vi "niFpga wdp fft DIF 16spc.vi"(0 "real data in":fxp<+/-,8,1>[](array[numeric])=[0.0, 0.0, 0.0, 0.0, 0.0, 0.0, 0.0, 0.0, 0.0, 0.0, 0.0, 0.0, 0.0, 0.0, 0.0, 0.0], 5 "imaginary data in":fxp<+/-,8,1>[](array[numeric])=[0.0, 0.0, 0.0, 0.0, 0.0, 0.0, 0.0, 0.0, 0.0, 0.0, 0.0, 0.0, 0.0, 0.0, 0.0, 0.0], 9 "input frame start":bool, 12 "enable":bool) -> (3 "data indices":u16[](array[numeric]), 4 "real data out":fxp<+,8,1>[](array[numeric]), 6 "imaginary data out":fxp<+,8,1>[](array[numeric]), 10 "output valid":bool, 14 "ready for frame":bool, 15 "output frame start":bool)   [LabVIEW 2017]
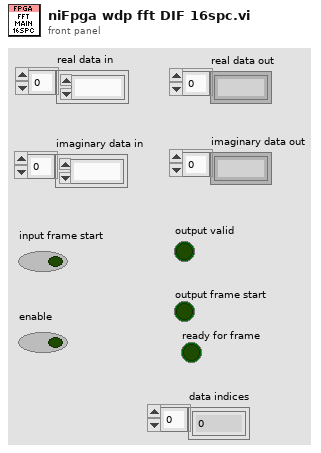
[diagram p1: front panel]
types:
  T1 = cluster{"internal input type":fxp<+/-,8,1>, "internal input type":fxp<+/-,8,1>}
  T2 = cluster{"internal input type":fxp<+/-,8,1>, "internal input type":fxp<+/-,8,1>}[]
  T3 = cluster{"x-y":fxp<+/-,20,13>, "x-y":fxp<+/-,20,13>}[]
  T4 = cluster{"data re":fxp<+/-,8,1>, "data im":fxp<+/-,8,1>}[]
  T5 = cluster{"data re":fxp<+/-,8,1>, "data im":fxp<+/-,8,1>}
  T6 = cluster{"twiddle factor type":fxp<+/-,16,2>, "twiddle factor type":fxp<+/-,16,2>}[]
  T7 = cluster{"x-y":fxp<+/-,19,12>, "x-y":fxp<+/-,19,12>}
  T8 = cluster{"x+y":fxp<+/-,19,12>, "x+y":fxp<+/-,19,12>}
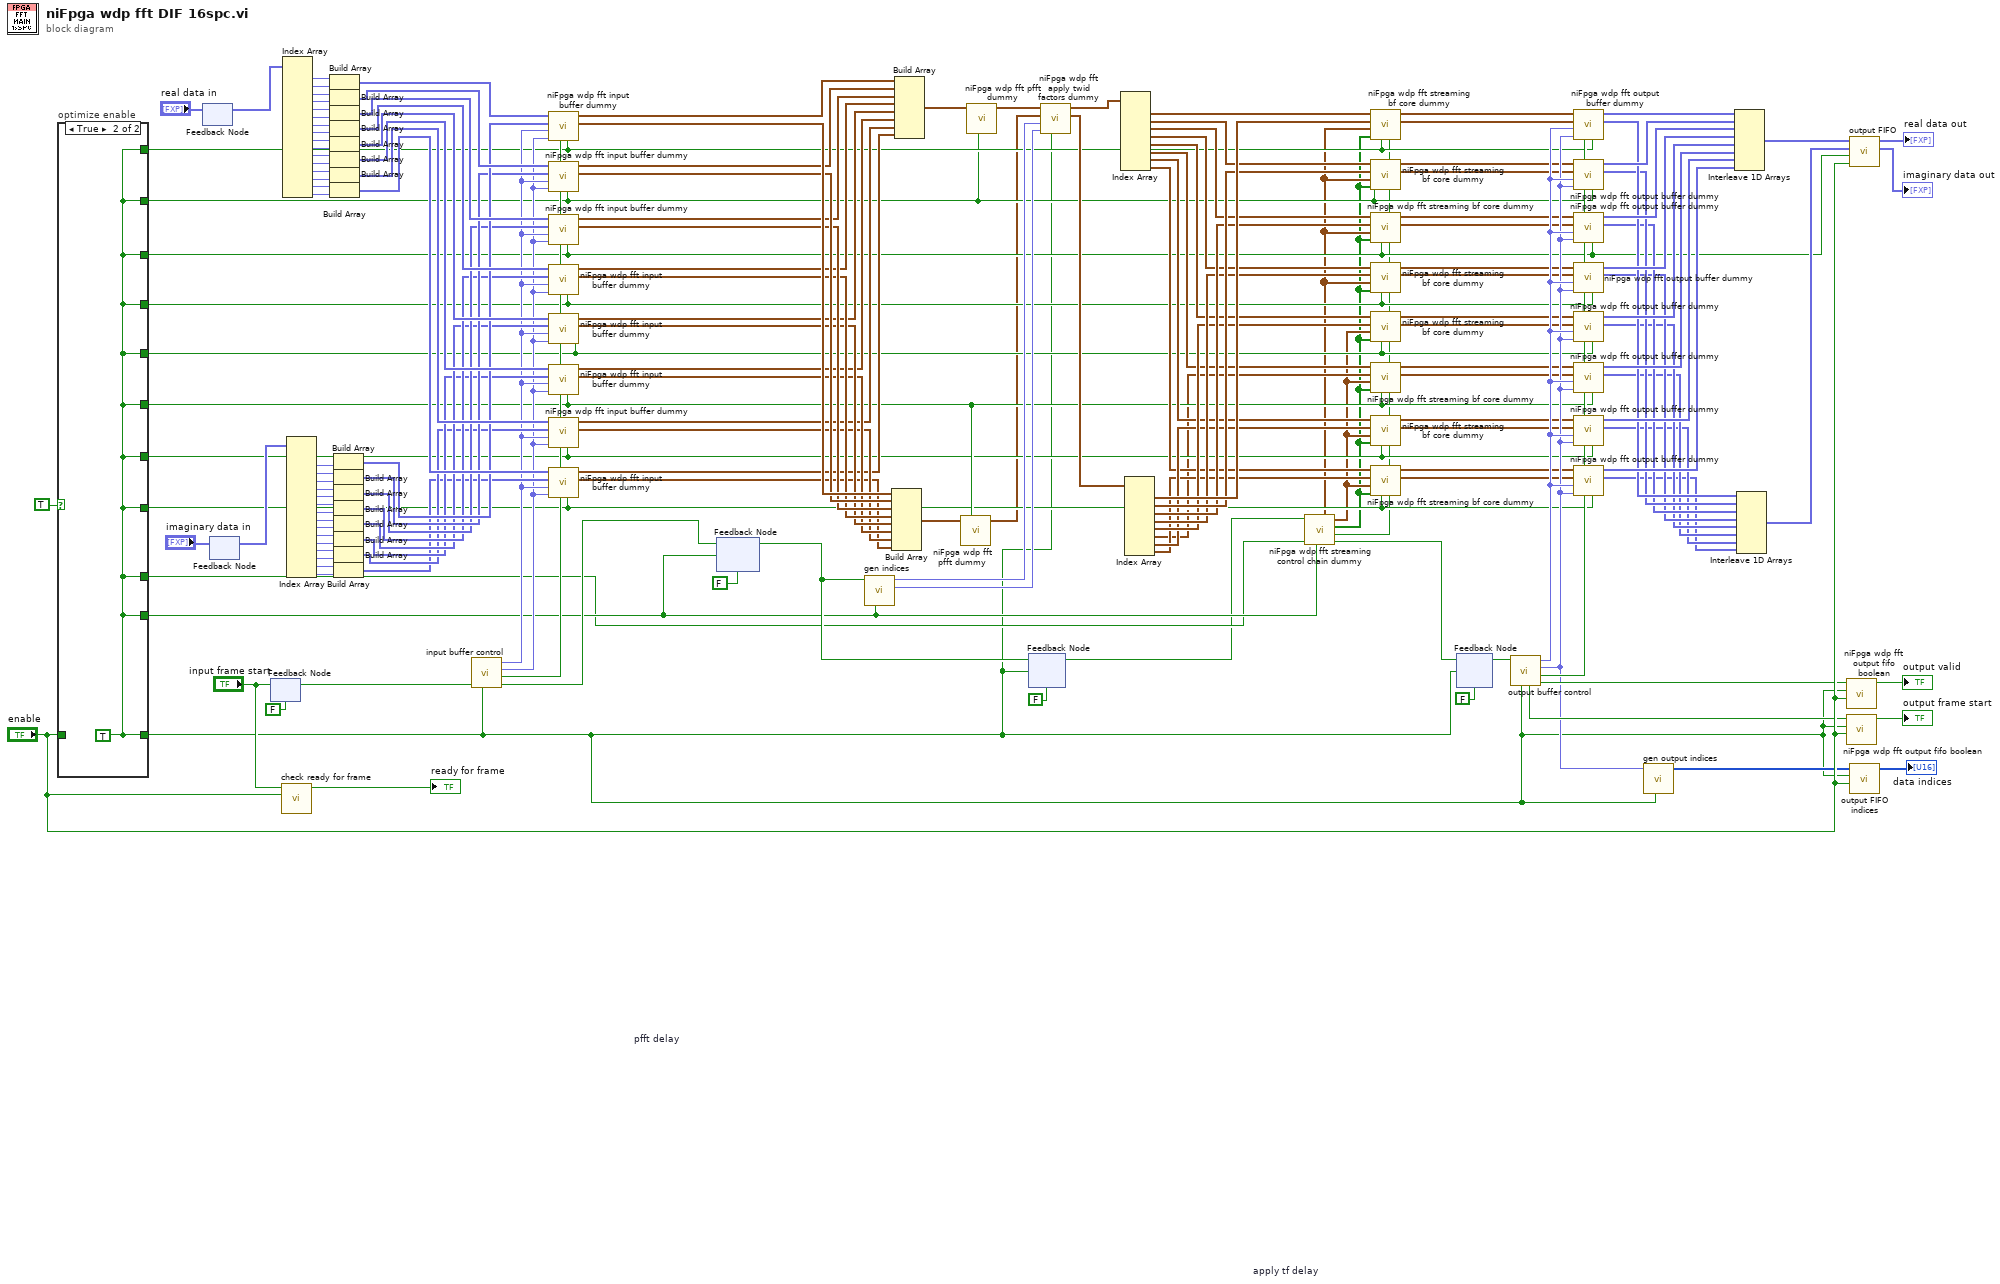
[diagram p0: block diagram]
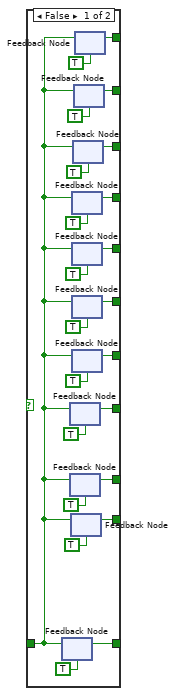
[diagram p2: hidden frame]
diagram:
  n1 = case "optimize enable" shown="True" TRUE {
    tunnel: [w191 w193] -> w41
    tunnel: [w189 w193] -> w45
    tunnel: [w180 w193] -> w57
    tunnel: [w179 w193] -> w56
    tunnel: [w178 w193] -> w55
    tunnel: [w177 w193] -> w54
    tunnel: [w176 w193] -> w53
    tunnel: [w175 w193] -> w52
    tunnel: [w174 w193] -> w51
    tunnel: [w173 w193] -> w50
    tunnel: "enable" -> [w171 _]
    tunnel: [w170 w193] -> w44
    frame False {
      n2 = feedback #1(TRUE ("enable")) -> (w191:bool)
      n3 = feedback-in #1(w171) -> ()
      n4 = feedback #2(TRUE ("enable")) -> (w173:bool)
      n5 = feedback-in #2(w171) -> ()
      n6 = feedback #3(TRUE ("enable")) -> (w170:bool)
      n7 = feedback-in #3(w171) -> ()
      n8 = feedback #4(TRUE ("enable")) -> (w189:bool)
      n9 = feedback-in #4(w171) -> ()
      n10 = feedback #5(TRUE ("enable")) -> (w177:bool)
      n11 = feedback-in #5(w171) -> ()
      n12 = feedback #6(TRUE ("enable")) -> (w176:bool)
      n13 = feedback-in #6(w171) -> ()
      n14 = feedback #7(TRUE ("enable")) -> (w175:bool)
      n15 = feedback-in #7(w171) -> ()
      n16 = feedback #8(TRUE ("enable")) -> (w174:bool)
      n17 = feedback-in #8(w171) -> ()
      n18 = feedback #9(TRUE ("enable")) -> (w178:bool)
      n19 = feedback-in #9(w171) -> ()
      n20 = feedback #10(TRUE ("enable")) -> (w179:bool)
      n21 = feedback-in #10(w171) -> ()
      n22 = feedback #11(TRUE ("enable")) -> (w180:bool)
      n23 = feedback-in #11(w171) -> ()
    }
    frame True {
      w193 = TRUE
    }
  }
  n24 = feedback #12() -> (w146:fxp<+/-,8,1>[])  [unwired: 1 in]
  n25 = feedback-in #12("real data in") -> ()
  n26 = feedback #13() -> (w137:fxp<+/-,8,1>[])  [unwired: 1 in]
  n27 = feedback-in #13("imaginary data in") -> ()
  n28 = feedback #14(FALSE ("enable")) -> (w164:bool)
  n29 = feedback-in #14("input frame start") -> ()
  n30 = call "check ready for frame"("enable"="enable", "frame start in"="input frame start") -> ("ready for frame"=→"ready for frame":bool)  [unwired: 9 in]
  n31 = Index Array(array=w146) -> (element #1=w39:fxp<+/-,8,1>, element #2=w38:fxp<+/-,8,1>, element #3=w37:fxp<+/-,8,1>, element #4=w36:fxp<+/-,8,1>, element #5=w35:fxp<+/-,8,1>, element #6=w34:fxp<+/-,8,1>, element #7=w33:fxp<+/-,8,1>, element #8=w32:fxp<+/-,8,1>, element #9=w31:fxp<+/-,8,1>, element #10=w30:fxp<+/-,8,1>, element #11=w29:fxp<+/-,8,1>, element #12=w28:fxp<+/-,8,1>, element #13=w27:fxp<+/-,8,1>, element #14=w26:fxp<+/-,8,1>, element #15=w25:fxp<+/-,8,1>, element #16=w24:fxp<+/-,8,1>)  [unwired: 16 in]
  n32 = Index Array(array=w137) -> (element #1=w8:fxp<+/-,8,1>, element #2=w9:fxp<+/-,8,1>, element #3=w10:fxp<+/-,8,1>, element #4=w11:fxp<+/-,8,1>, element #5=w12:fxp<+/-,8,1>, element #6=w13:fxp<+/-,8,1>, element #7=w14:fxp<+/-,8,1>, element #8=w15:fxp<+/-,8,1>, element #9=w16:fxp<+/-,8,1>, element #10=w17:fxp<+/-,8,1>, element #11=w18:fxp<+/-,8,1>, element #12=w19:fxp<+/-,8,1>, element #13=w20:fxp<+/-,8,1>, element #14=w21:fxp<+/-,8,1>, element #15=w22:fxp<+/-,8,1>, element #16=w23:fxp<+/-,8,1>)  [unwired: 16 in]
  n33 = Build Array(w39, w38) -> (w145:fxp<+/-,8,1>[])
  n34 = Build Array(w37, w36) -> (w144:fxp<+/-,8,1>[])
  n35 = Build Array(w35, w34) -> (w143:fxp<+/-,8,1>[])
  n36 = Build Array(w33, w32) -> (w142:fxp<+/-,8,1>[])
  n37 = Build Array(w31, w30) -> (w141:fxp<+/-,8,1>[])
  n38 = Build Array(w29, w28) -> (w140:fxp<+/-,8,1>[])
  n39 = Build Array(w27, w26) -> (w139:fxp<+/-,8,1>[])
  n40 = Build Array(w25, w24) -> (w138:fxp<+/-,8,1>[])
  n41 = Build Array(w8, w9) -> (w136:fxp<+/-,8,1>[])
  n42 = Build Array(w10, w11) -> (w135:fxp<+/-,8,1>[])
  n43 = Build Array(w12, w13) -> (w134:fxp<+/-,8,1>[])
  n44 = Build Array(w14, w15) -> (w133:fxp<+/-,8,1>[])
  n45 = Build Array(w16, w17) -> (w132:fxp<+/-,8,1>[])
  n46 = Build Array(w18, w19) -> (w131:fxp<+/-,8,1>[])
  n47 = Build Array(w20, w21) -> (w130:fxp<+/-,8,1>[])
  n48 = Build Array(w22, w23) -> (w129:fxp<+/-,8,1>[])
  n49 = call "input buffer control"("enable"=w41, "frame start in"=w164) -> ("frame start out"=w88:bool, "write memory 2?"=w121:bool, "read index"=w127:fxp<+,9,9>, "write index"=w128:fxp<+,8,8>)  [unwired: 6 in]
  n50 = call <vilib>:"niFpga wdp fft input buffer dummy.vi"("enable"=w57, "write memory 2?"=w121, "read index"=w127, "write index"=w128, "data in im"=w136, "data in re"=w145) -> ("data out 1"=w107:T1, "data out 0"=w108:T1)  [unwired: 4 in]
  n51 = call <vilib>:"niFpga wdp fft input buffer dummy.vi"("enable"=w56, "write memory 2?"=w121, "read index"=w127, "write index"=w128, "data in im"=w135, "data in re"=w144) -> ("data out 1"=w105:T1, "data out 0"=w106:T1)  [unwired: 4 in]
  n52 = call <vilib>:"niFpga wdp fft input buffer dummy.vi"("enable"=w55, "write memory 2?"=w121, "read index"=w127, "write index"=w128, "data in im"=w134, "data in re"=w143) -> ("data out 1"=w103:T1, "data out 0"=w104:T1)  [unwired: 4 in]
  n53 = call <vilib>:"niFpga wdp fft input buffer dummy.vi"("enable"=w54, "write memory 2?"=w121, "read index"=w127, "write index"=w128, "data in im"=w133, "data in re"=w142) -> ("data out 1"=w101:T1, "data out 0"=w102:T1)  [unwired: 4 in]
  n54 = call <vilib>:"niFpga wdp fft input buffer dummy.vi"("enable"=w53, "write memory 2?"=w121, "read index"=w127, "write index"=w128, "data in im"=w132, "data in re"=w141) -> ("data out 1"=w99:T1, "data out 0"=w100:T1)  [unwired: 4 in]
  n55 = call <vilib>:"niFpga wdp fft input buffer dummy.vi"("enable"=w52, "write memory 2?"=w121, "read index"=w127, "write index"=w128, "data in im"=w131, "data in re"=w140) -> ("data out 1"=w97:T1, "data out 0"=w98:T1)  [unwired: 4 in]
  n56 = call <vilib>:"niFpga wdp fft input buffer dummy.vi"("enable"=w51, "write memory 2?"=w121, "read index"=w127, "write index"=w128, "data in im"=w130, "data in re"=w139) -> ("data out 1"=w95:T1, "data out 0"=w96:T1)  [unwired: 4 in]
  n57 = call <vilib>:"niFpga wdp fft input buffer dummy.vi"("enable"=w50, "write memory 2?"=w121, "read index"=w127, "write index"=w128, "data in im"=w129, "data in re"=w138) -> ("data out 1"=w93:T1, "data out 0"=w94:T1)  [unwired: 4 in]
  n58 = feedback #15 "pfft delay"(FALSE) -> (w46:bool)
  n59 = feedback-in #15(w88, w45) -> ()
  n60 = call "gen indices"("enable"=w45, "frame start"=w46) -> ("data index 1"=w89:fxp<+,10,10>, "data index 0"=w90:fxp<+,10,10>)  [unwired: 8 in]
  n61 = Build Array(w107, w105, w103, w101, w99, w97, w95, w93) -> (w92:T2)
  n62 = Build Array(w108, w106, w104, w102, w100, w98, w96, w94) -> (w111:T2)
  n63 = call <vilib>:"niFpga wdp fft pfft dummy.vi"("enable"=w52, "data in"=w92) -> ("data out"=w5:T3)  [unwired: 9 in]
  n64 = call <vilib>:"niFpga wdp fft pfft dummy.vi"("enable"=w56, "data in"=w111) -> ("data out"=w6:T3)  [unwired: 9 in]
  n65 = feedback #16 "apply tf delay"(FALSE) -> (w40:bool)
  n66 = feedback-in #16(w46, w41) -> ()
  n67 = call <vilib>:"niFpga wdp fft apply twid factors dummy.vi"("enable"=w41, "data index 1"=w89, "data index 0"=w90, "data in 1"=w5, "data in 0"=w6) -> ("data out 1"=w109:T4, "data out 0"=w110:T4)  [unwired: 5 in]
  n68 = Index Array(array=w110) -> (element #1=w87:T5, element #2=w83:T5, element #3=w79:T5, element #4=w75:T5, element #5=w71:T5, element #6=w67:T5, element #7=w65:T5, element #8=w61:T5)  [unwired: 8 in]
  n69 = Index Array(array=w109) -> (element #1=w85:T5, element #2=w81:T5, element #3=w77:T5, element #4=w73:T5, element #5=w70:T5, element #6=w49:T5, element #7=w63:T5, element #8=w59:T5)  [unwired: 8 in]
  n70 = call <vilib>:"niFpga wdp fft streaming control chain dummy.vi"("enable"=w45, "enable 1"=w44, "input frame start"=w40) -> ("frame start"=w43:bool, "index=0?"=w4:bool, "switch"=w1:bool[], "twiddle factors 1"=w2:T6, "twiddle factors"=w3:T6)  [unwired: 4 in]
  n71 = call <vilib>:"niFpga wdp fft streaming bf core dummy.vi"("index=0?"=w4, "enable"=w57, "switch"=w1, "twiddle factors"=w3, "data in 1"=w85, "data in 0"=w87) -> ("data out 1"=w84:T7, "data out 0"=w86:T8)  [unwired: 4 in]
  n72 = call <vilib>:"niFpga wdp fft streaming bf core dummy.vi"("index=0?"=w4, "enable"=w56, "switch"=w1, "twiddle factors"=w3, "data in 1"=w81, "data in 0"=w83) -> ("data out 1"=w80:T7, "data out 0"=w82:T8)  [unwired: 4 in]
  n73 = call <vilib>:"niFpga wdp fft streaming bf core dummy.vi"("index=0?"=w4, "enable"=w55, "switch"=w1, "twiddle factors"=w3, "data in 1"=w77, "data in 0"=w79) -> ("data out 1"=w76:T7, "data out 0"=w78:T8)  [unwired: 4 in]
  n74 = call <vilib>:"niFpga wdp fft streaming bf core dummy.vi"("index=0?"=w4, "enable"=w54, "switch"=w1, "twiddle factors"=w3, "data in 1"=w73, "data in 0"=w75) -> ("data out 1"=w72:T7, "data out 0"=w74:T8)  [unwired: 4 in]
  n75 = call <vilib>:"niFpga wdp fft streaming bf core dummy.vi"("index=0?"=w4, "enable"=w53, "switch"=w1, "twiddle factors"=w2, "data in 1"=w70, "data in 0"=w71) -> ("data out 1"=w68:T7, "data out 0"=w69:T8)  [unwired: 4 in]
  n76 = call <vilib>:"niFpga wdp fft streaming bf core dummy.vi"("index=0?"=w4, "enable"=w52, "switch"=w1, "twiddle factors"=w2, "data in 1"=w49, "data in 0"=w67) -> ("data out 1"=w48:T7, "data out 0"=w66:T8)  [unwired: 4 in]
  n77 = call <vilib>:"niFpga wdp fft streaming bf core dummy.vi"("index=0?"=w4, "enable"=w51, "switch"=w1, "twiddle factors"=w2, "data in 1"=w63, "data in 0"=w65) -> ("data out 1"=w62:T7, "data out 0"=w64:T8)  [unwired: 4 in]
  n78 = call <vilib>:"niFpga wdp fft streaming bf core dummy.vi"("index=0?"=w4, "enable"=w50, "switch"=w1, "twiddle factors"=w2, "data in 1"=w59, "data in 0"=w61) -> ("data out 1"=w58:T7, "data out 0"=w60:T8)  [unwired: 4 in]
  n79 = feedback #17 ("delay")(FALSE) -> (w42:bool)
  n80 = feedback-in #17(w43, w41) -> ()
  n81 = call "output buffer control"("enable"=w41, "frame start"=w42) -> ("output valid?"=w117:bool, "memory switch"=w114:bool, "read index"=w113:fxp<+,4,4>, "write index"=w115:fxp<+,9,9>, "frame start?"=w116:bool)  [unwired: 5 in]
  n82 = call <vilib>:"niFpga wdp fft output buffer dummy.vi"("enable"=w57, "memory switch"=w114, "read index"=w113, "write index"=w115, "data in 1"=w84, "data in 0"=w86) -> ("data out im"=w154:fxp<+/-,32,16>[], "data out re"=w162:fxp<+/-,32,16>[])  [unwired: 4 in]
  n83 = call <vilib>:"niFpga wdp fft output buffer dummy.vi"("enable"=w56, "memory switch"=w114, "read index"=w113, "write index"=w115, "data in 1"=w80, "data in 0"=w82) -> ("data out im"=w153:fxp<+/-,32,16>[], "data out re"=w161:fxp<+/-,32,16>[])  [unwired: 4 in]
  n84 = call <vilib>:"niFpga wdp fft output buffer dummy.vi"("enable"=w55, "memory switch"=w114, "read index"=w113, "write index"=w115, "data in 1"=w76, "data in 0"=w78) -> ("data out im"=w152:fxp<+/-,32,16>[], "data out re"=w160:fxp<+/-,32,16>[])  [unwired: 4 in]
  n85 = call <vilib>:"niFpga wdp fft output buffer dummy.vi"("enable"=w54, "memory switch"=w114, "read index"=w113, "write index"=w115, "data in 1"=w72, "data in 0"=w74) -> ("data out im"=w151:fxp<+/-,32,16>[], "data out re"=w159:fxp<+/-,32,16>[])  [unwired: 4 in]
  n86 = call <vilib>:"niFpga wdp fft output buffer dummy.vi"("enable"=w53, "memory switch"=w114, "read index"=w113, "write index"=w115, "data in 1"=w68, "data in 0"=w69) -> ("data out im"=w150:fxp<+/-,32,16>[], "data out re"=w158:fxp<+/-,32,16>[])  [unwired: 4 in]
  n87 = call <vilib>:"niFpga wdp fft output buffer dummy.vi"("enable"=w52, "memory switch"=w114, "read index"=w113, "write index"=w115, "data in 1"=w48, "data in 0"=w66) -> ("data out im"=w149:fxp<+/-,32,16>[], "data out re"=w157:fxp<+/-,32,16>[])  [unwired: 4 in]
  n88 = call <vilib>:"niFpga wdp fft output buffer dummy.vi"("enable"=w51, "memory switch"=w114, "read index"=w113, "write index"=w115, "data in 1"=w62, "data in 0"=w64) -> ("data out im"=w148:fxp<+/-,32,16>[], "data out re"=w156:fxp<+/-,32,16>[])  [unwired: 4 in]
  n89 = call <vilib>:"niFpga wdp fft output buffer dummy.vi"("enable"=w50, "memory switch"=w114, "read index"=w113, "write index"=w115, "data in 1"=w58, "data in 0"=w60) -> ("data out im"=w147:fxp<+/-,32,16>[], "data out re"=w155:fxp<+/-,32,16>[])  [unwired: 4 in]
  n90 = call "gen output indices"("enable"=w41, "index"=w113) -> ("data indices"=w112:u16[])  [unwired: 9 in]
  n91 = Interleave 1D Arrays(w162, w161, w160, w159, w158, w157, w156, w155) -> (w125:fxp<+/-,32,16>[])
  n92 = Interleave 1D Arrays(w154, w153, w152, w151, w150, w149, w148, w147) -> (w123:fxp<+/-,32,16>[])
  n93 = call <vilib>:"niFpga wdp fft output fifo boolean.vi"("enable"="enable", "enable with delay"=w41, "boolean in"=w117) -> ("boolean out"=→"output valid":bool)  [unwired: 8 in]
  n94 = call <vilib>:"niFpga wdp fft output fifo boolean.vi"("enable"="enable", "enable with delay"=w41, "boolean in"=w116) -> ("boolean out"=→"output frame start":bool)  [unwired: 8 in]
  n95 = call "output FIFO"("enable"="enable", "enable with delay"=w55, "data in 1"=w123, "data in 0"=w125) -> ("data out 1"=→"imaginary data out":fxp<+,8,1>[], "data out 0"=→"real data out":fxp<+,8,1>[])  [unwired: 6 in]
  n96 = call "output FIFO indices"("enable"="enable", "enable with delay"=w41, "data in"=w112) -> ("data out"=→"data indices":u16[])  [unwired: 8 in]
